vi "DataReceiver.vi"() -> ()   [LabVIEW 2013]
panel:
  out "Waveform Graph":sgl[][](graph)
  in  "Stop":bool
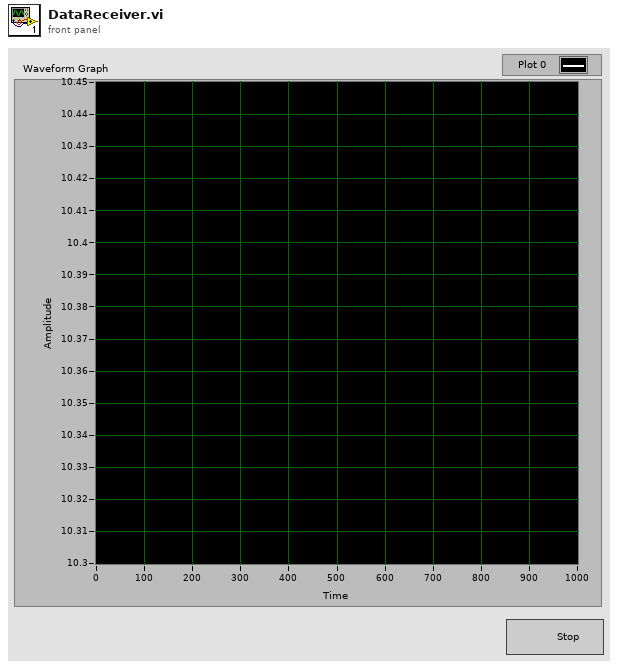
[diagram p1: front panel]
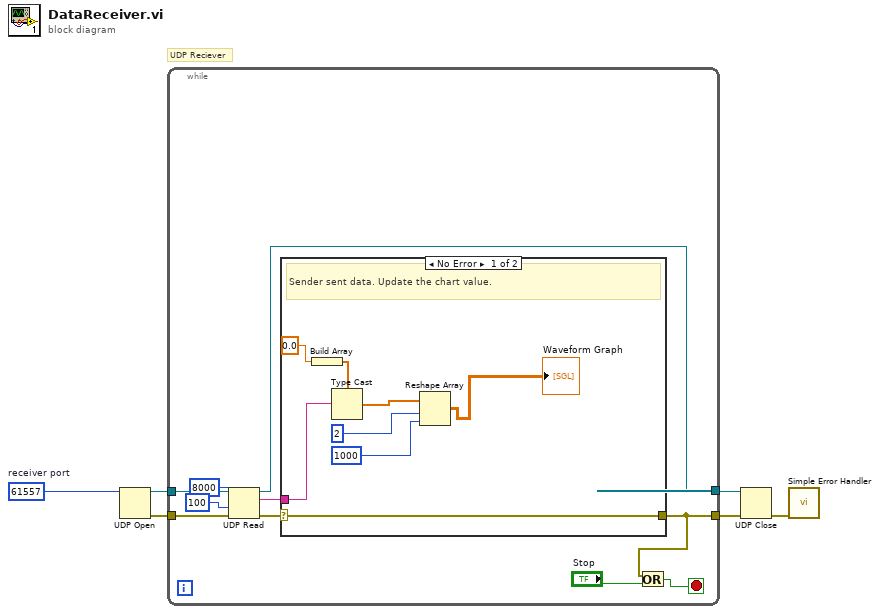
[diagram p0: block diagram]
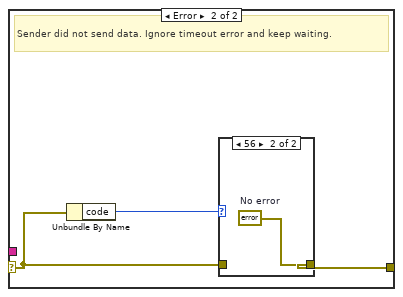
[diagram p2: hidden frame]
diagram:
  w5 = u16 61557  # receiver port
  # "UDP Reciever"
  n1 = UDP Open(11:w5) -> (port=w2:refnum<k16>, 0:w1:errorcluster)  [unwired: 4 in, 1 out]
  n2 = while {
    tunnel: [w10] -> w4
    tunnel: [w12] -> w3
    tunnel: w2 -> [w11]
    tunnel: w1 -> [w8]
    stop <- w9 stop-if-true
    n3 = UDP Read(connection ID=w11, max size (548)=8000, timeout ms (25000)=100, 8:w8) -> (data out=w14:string, error out=w13:errorcluster, 3:w12:refnum<k16>)  [unwired: 2 out]
    n4 = case shown="No Error" w13 {
      selector: w13 -> [w24 w26]
      tunnel: w14 -> [w23 _]
      tunnel: [w24 w25] -> w10
      frame No Error {
        # "Sender sent data. Update the chart value."
        n5 = Build Array(sgl 0.0) -> (w18:sgl[])
        n6 = Type Cast(type=w18, x=w23) -> (*(type *) &x=w22:sgl[])
        n7 = Reshape Array(w22, 2 ("dimension size"), 1000 ("dimension size")) -> (→"Waveform Graph":sgl[][])
      }
      frame Error {
        # "Sender did not send data. Ignore timeout error and keep waiting."
        n8 = Unbundle By Name(w26) -> ("code"=w27:i32)
        n9 = case shown="56" w27 {
          tunnel: w26 -> [w28 _]
          tunnel: [w28 w29] -> w25
          frame Default {
          }
          frame 56 {
            w29 = errorcluster {"status"=FALSE, "code"=0, "source"=""}  # No error
          }
        }
      }
    }
    n10 = Or(x=w10, y="Stop") -> (x .or. y?=w9:bool)
  }
  n11 = UDP Close(connection ID=w3, 8:w4) -> (error out=w6:errorcluster)  [unwired: 1 out]
  n12 = call <vilib>:"Simple Error Handler.vi"("error in (no error)"=w6) -> ()  [unwired: 1 in, 8 out]
